vi "main.vi"() -> ()   [LabVIEW 2017]
panel:
  in  "选项卡控件":enum32{"CONTROL", "选项卡 2"}(tab)
  in  "VISA资源名称":refnum<visa-resource-name>
  in  "增益选择":u16(ring) items=["±6.144V", "±4.096V", "±2.048V", "±1.024V", "±0.512V", "±0.256V"]
  in  "连接方式":u16(ring) items=["Serial", "WiFi", "Dual"]
  in  "Interval_ms":dbl
  in  "连接":bool
  in  "?":bool
  in  "停止":bool
  out "数值显示控件 37":dbl
  out "数值显示控件":dbl
  out "数值显示控件 2":dbl
  out "数值显示控件 3":dbl
  out "数值显示控件 4":dbl
  out "数值显示控件 5":dbl
  out "数值显示控件 6":dbl
  out "数值显示控件 7":dbl
  out "数值显示控件 8":dbl
  out "数值显示控件 9":dbl
  out "数值显示控件 10":dbl
  out "数值显示控件 11":dbl
  out "数值显示控件 12":dbl
  out "数值显示控件 13":dbl
  out "数值显示控件 14":dbl
  out "数值显示控件 15":dbl
  out "数值显示控件 16":dbl
  out "数值显示控件 17":dbl
  out "数值显示控件 18":dbl
  out "数值显示控件 19":dbl
  out "数值显示控件 20":dbl
  out "数值显示控件 21":dbl
  out "数值显示控件 22":dbl
  out "数值显示控件 23":dbl
  out "数值显示控件 24":dbl
  out "数值显示控件 25":dbl
  out "数值显示控件 26":dbl
  out "数值显示控件 27":dbl
  out "数值显示控件 28":dbl
  out "数值显示控件 29":dbl
  out "数值显示控件 30":dbl
  out "数值显示控件 31":dbl
  out "数值显示控件 32":dbl
  out "数值显示控件 33":dbl
  out "数值显示控件 34":dbl
  out "数值显示控件 35":dbl
  out "数值显示控件 36":dbl
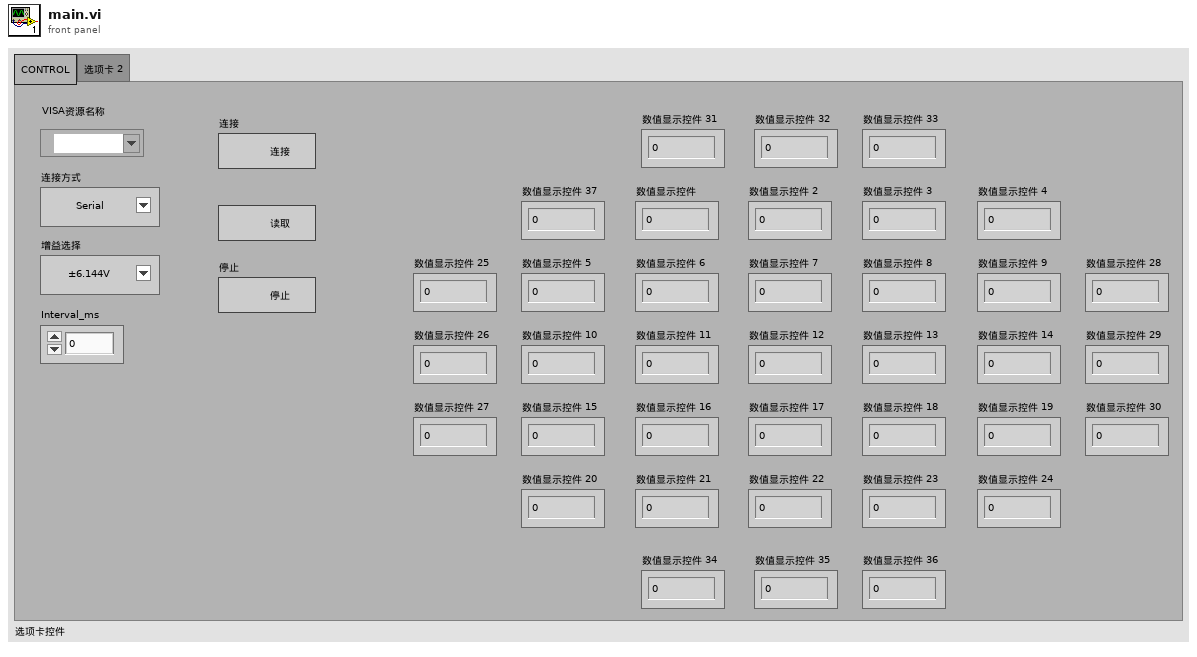
[diagram p1: front panel]
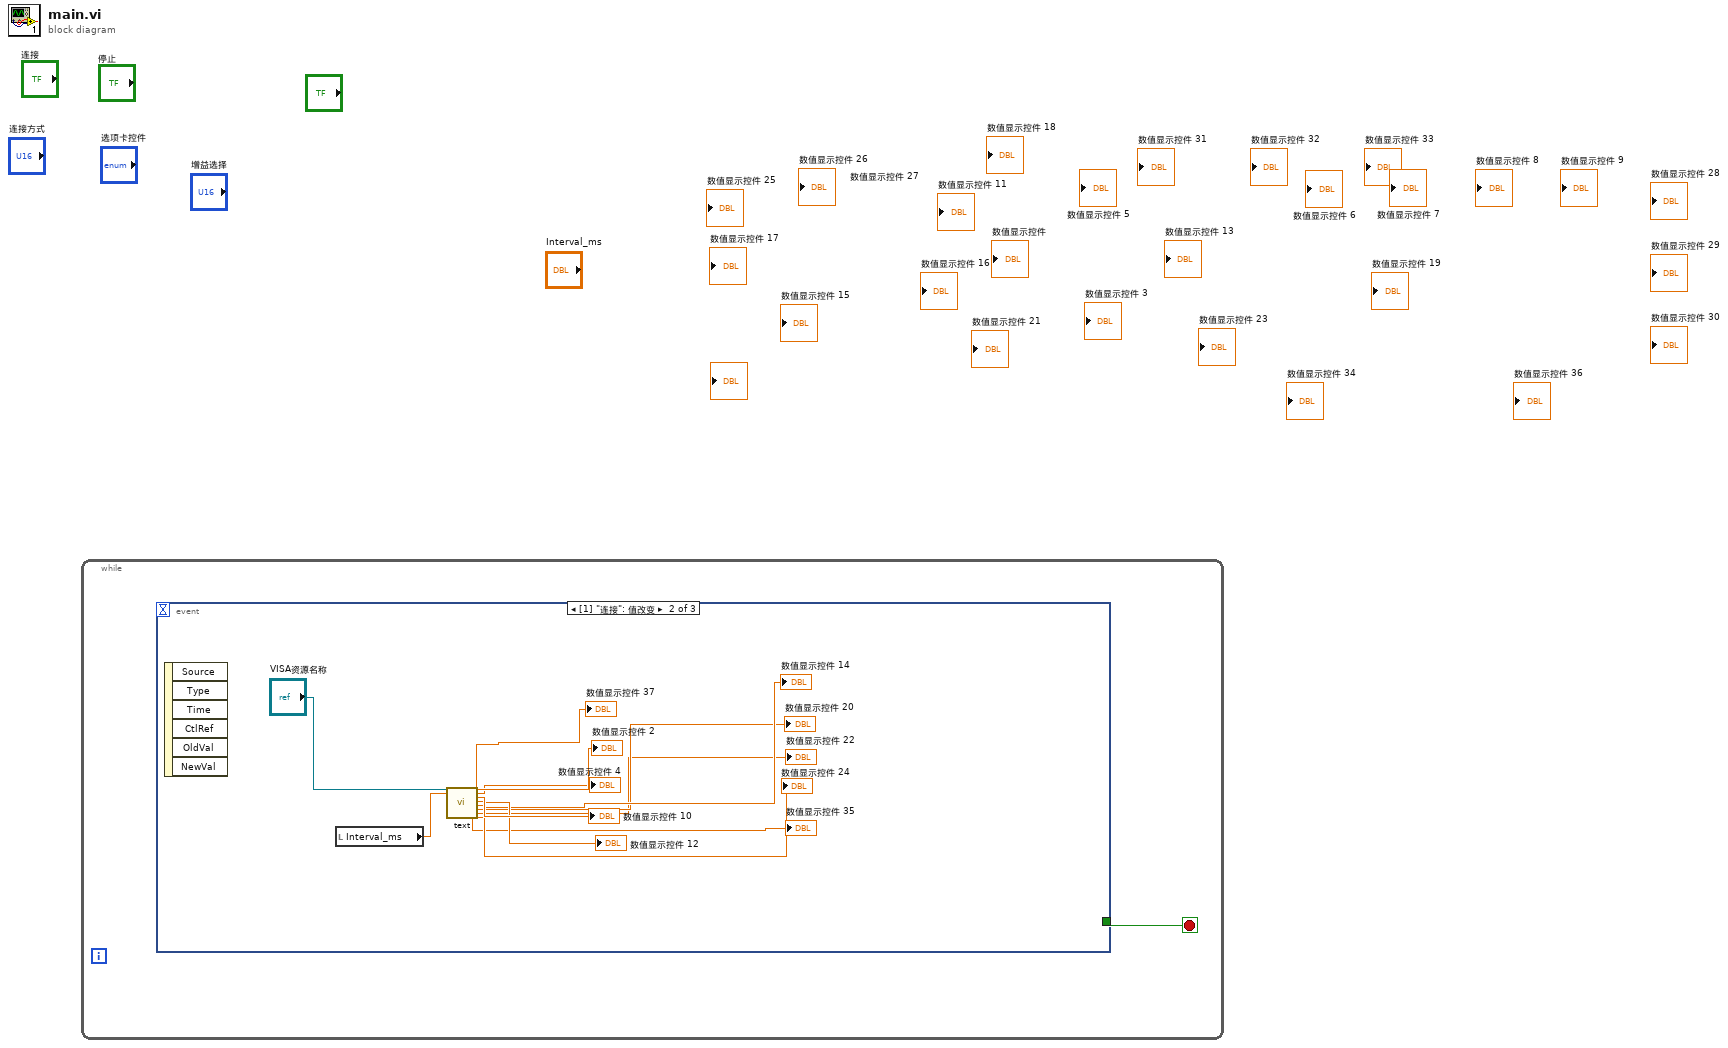
[diagram p0: block diagram]
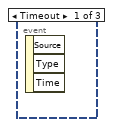
[diagram p2: hidden frame]
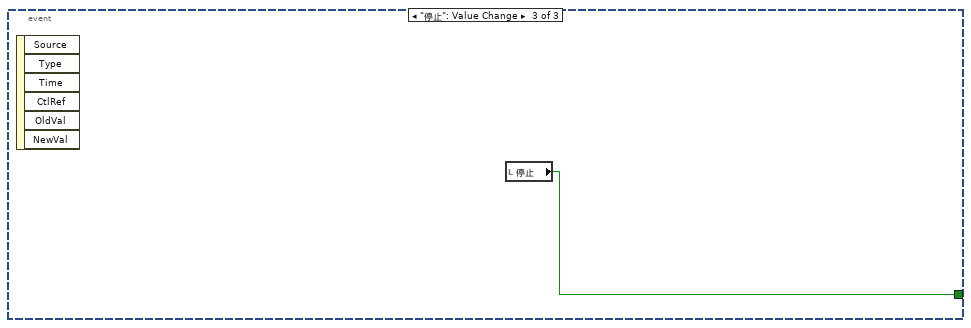
[diagram p3: hidden frame]
diagram:
  n1 = while {
    stop <- w1 stop-if-true
    n2 = event shown="[1] \"连接\": 值改变" {
      selector: _ -> [_ _ _]
      dyn-events: _ -> [_ _ _]
      timeout: _ -> [_ _ _]
      tunnel: [_ _ w13] -> w1
      event Timeout {
        n3 = event-data() -> ()  [unwired: 1 in, 3 out]
      }
      event "连接": Value Change {
        n4 = event-data() -> ()  [unwired: 1 in, 6 out]
        n5 = local read "Interval_ms"() -> (w11:dbl)
        n6 = call "text.vi"("VISA资源名称 2"="VISA资源名称", "读取速率"=w11) -> ("值 10"=→"数值显示控件 35":dbl, "值"=→"数值显示控件 37" →"数值显示控件 2":dbl, "值 3"=→"数值显示控件 4":dbl, "值 4"=→"数值显示控件 10":dbl, "值 5"=→"数值显示控件 12":dbl, "值 6"=→"数值显示控件 14":dbl, "值 7"=→"数值显示控件 20":dbl, "值 8"=→"数值显示控件 22":dbl, "值 9"=→"数值显示控件 24":dbl)  [unwired: 17 in]
      }
      event "停止": Value Change {
        n7 = event-data() -> ()  [unwired: 1 in, 6 out]
        n8 = local read "停止"() -> (w13:bool)
      }
    }
  }
